vi "Data Save0.vi"(8 "error in (no error)":errorcluster caption="Error In", 10 "Path":path, 11 "Data":variant) -> (0 "error out":errorcluster caption="Error Out")   [LabVIEW 2020]
uses:
  <vilib>/Analysis/baseanly.llb/Mean (DBL).vi
  <vilib>/Utility/file.llb/Write Delimited Spreadsheet (string).vi
  <vilib>/Analysis/NI_AALBase.lvlib
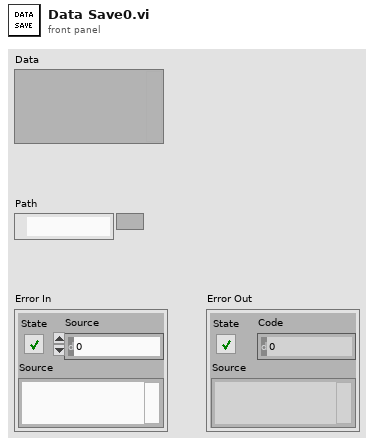
[diagram p1: front panel]
types:
  T1 = cluster{"Name":string, "Data":cluster{"Time":string, "Data":string}[]}
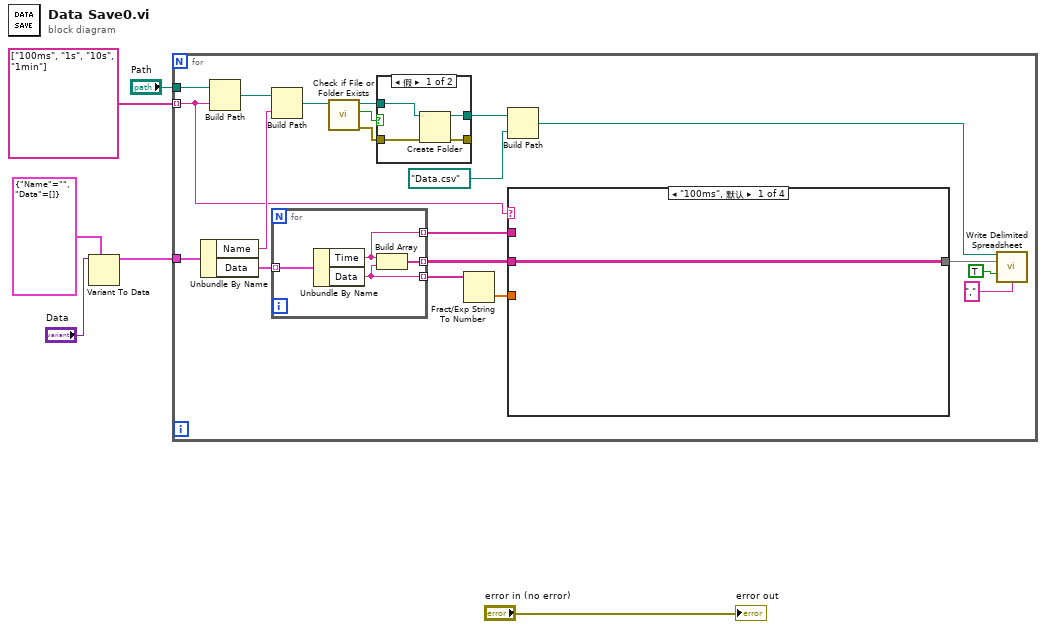
[diagram p0: block diagram]
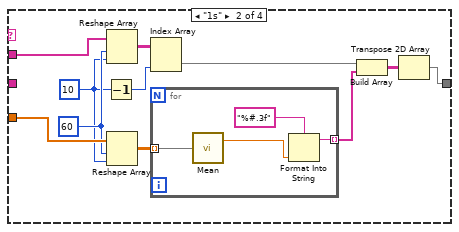
[diagram p2: hidden frame]
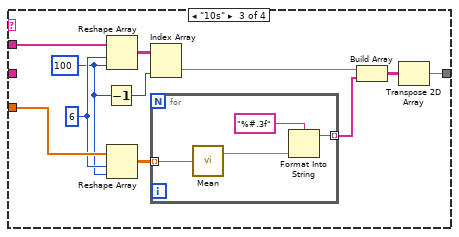
[diagram p3: hidden frame]
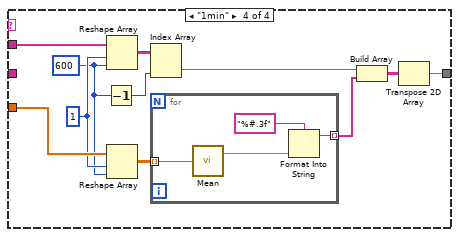
[diagram p4: hidden frame]
diagram:
  n1 = Variant To Data(type=T1 {"Name"="", "Data"=[]} ("输出簇"), Variant="Data") -> (data=w2:T1)  [unwired: 1 in, 1 out]
  n2 = for {
    tunnel: w2 -> [w26]
    tunnel: "Path" -> [w14]
    tunnel: string[] ["100ms", "1s", "10s", "1min"] ("名称或相对路径") -> [w13] mode=indexing
    n3 = Unbundle By Name(w26) -> ("Name"=w15:string, "Data"=w12:cluster{"Time":string, "Data":string}[])
    n4 = Build Path(base path=w14, name or relative path=w13) -> (appended path=w18:path)
    n5 = Build Path(base path=w18, name or relative path=w15) -> (appended path=w17:path)
    n6 = for {
      tunnel: w12 -> [w30] mode=indexing
      tunnel: [w29] -> w11 mode=indexing
      tunnel: [w28] -> w9 mode=indexing
      tunnel: [w27] -> w7 mode=indexing
      n7 = Unbundle By Name(w30) -> ("Time"=w27:string, "Data"=w28:string)
      n8 = Build Array(w27, w28) -> (w29:string[])
    }
    n9 = call <vilib>:"Check if File or Folder Exists.vi"("path"=w17) -> ("error out"=w21:errorcluster, "file or folder exists?"=w20:bool, "dup path"=w22:path)  [unwired: 8 in]
    n10 = case shown="假" w20 {
      tunnel: w22 -> [w80 w82]
      tunnel: w21 -> [w79 w81]
      tunnel: [w78 w82] -> w19
      tunnel: [w77 w81] -> _
      frame False {
        n11 = Create Folder(path (use dialog)=w80, error in=w79) -> (created path=w78:path, error out=w77:errorcluster)  [unwired: 1 in, 1 out]
      }
      frame True {
      }
    }
    n12 = Fract/Exp String To Number(string=w9) -> (number=w8:dbl[])  [unwired: 3 in, 1 out]
    n13 = Build Path(base path=w19, name or relative path=path "Data.csv" ("名称或相对路径")) -> (appended path=w25:path)
    n14 = case shown="\"100ms\", 默认" w13 {
      tunnel: w11 -> [w31 _ _ _]
      tunnel: [w31 w38 w53 w68] -> w10
      tunnel: w8 -> [_ w42 w57 w72]
      tunnel: w7 -> [_ w37 w52 w67]
      frame "100ms", Default {
      }
      frame "1s" {
        w33 = 10 ("维数大小")
        w36 = 60 ("维数大小")
        n15 = Decrement(x=w33) -> (x-1=w32:i32)
        n16 = Reshape Array(w37, w36, w33) -> (w35:string[][])
        n17 = Reshape Array(w42, w36, w33) -> (w41:dbl[][])
        n18 = Index Array(array=w35, index (col)=w32) -> (element=w34:string[])  [unwired: 1 in]
        n19 = for {
          tunnel: w41 -> [w46] mode=indexing
          tunnel: [w43] -> w40 mode=indexing
          n20 = call-poly <vilib>:"Mean.vi"("X"=w46) -> ("mean"=w44:dbl)  [unwired: 1 out]
          n21 = Format Into String(format string="%#.3f" ("格式字符串"), w44) -> (resulting string=w43:string)  [unwired: 2 in, 1 out]
        }
        n22 = Build Array(w34, w40) -> (w39:string[][])
        n23 = Transpose 2D Array(2D array=w39) -> (transposed array=w38:string[][])
      }
      frame "10s" {
        w48 = 100 ("维数大小")
        w51 = 6 ("维数大小")
        n24 = Decrement(x=w48) -> (x-1=w47:i32)
        n25 = Reshape Array(w52, w51, w48) -> (w50:string[][])
        n26 = Reshape Array(w57, w51, w48) -> (w56:dbl[][])
        n27 = Index Array(array=w50, index (col)=w47) -> (element=w49:string[])  [unwired: 1 in]
        n28 = for {
          tunnel: w56 -> [w61] mode=indexing
          tunnel: [w58] -> w55 mode=indexing
          n29 = call-poly <vilib>:"Mean.vi"("X"=w61) -> ("mean"=w59:dbl)  [unwired: 1 out]
          n30 = Format Into String(format string="%#.3f" ("格式字符串"), w59) -> (resulting string=w58:string)  [unwired: 2 in, 1 out]
        }
        n31 = Build Array(w49, w55) -> (w54:string[][])
        n32 = Transpose 2D Array(2D array=w54) -> (transposed array=w53:string[][])
      }
      frame "1min" {
        w63 = 600 ("维数大小")
        w66 = 1 ("维数大小")
        n33 = Decrement(x=w63) -> (x-1=w62:i32)
        n34 = Reshape Array(w67, w66, w63) -> (w65:string[][])
        n35 = Reshape Array(w72, w66, w63) -> (w71:dbl[][])
        n36 = Index Array(array=w65, index (col)=w62) -> (element=w64:string[])  [unwired: 1 in]
        n37 = for {
          tunnel: w71 -> [w76] mode=indexing
          tunnel: [w73] -> w70 mode=indexing
          n38 = call-poly <vilib>:"Mean.vi"("X"=w76) -> ("mean"=w74:dbl)  [unwired: 1 out]
          n39 = Format Into String(format string="%#.3f" ("格式字符串"), w74) -> (resulting string=w73:string)  [unwired: 2 in, 1 out]
        }
        n40 = Build Array(w64, w70) -> (w69:string[][])
        n41 = Transpose 2D Array(2D array=w69) -> (transposed array=w68:string[][])
      }
    }
    n42 = call-poly <vilib>:"Write Delimited Spreadsheet.vi"("file path (dialog if empty)"=w25, "2D data"=w10, "append to file? (new file:F)"=TRUE, "delimiter (\\t)"="," ("delimiter (\\t)")) -> ()  [unwired: 10 in, 2 out]
  }
  "error out" <- "error in (no error)"
